vi "seriellTest.vi"() -> ()   [LabVIEW 2017]
uses:
  <vilib>/Utility/error.llb/Error Cluster From Error Code.vi
  <vilib>/rvi/errors/niLvFpgaAdjustHostInterfaceError.vi
  <vilib>/FPGAPlugInAG/cRIO-9035/niLvFpga_Close_cRIO-9035.vi
  <vilib>/rvi/interface/nirviMethod/nirviMethod.xnode
  FPGA Bitfiles/HAGAR-V_FPGATargetECD_FPGA-ProgrammECD_LbBtUh8SPQY.lvbitx
  FPGA_ECD/FPGA-Programm_ECD.vi
  <vilib>/rvi/interface/nirviReadWriteControl/nirviReadWriteControl.xnode
  <vilib>/rvi/interface/nirviCloseFPGA/nirviCloseFPGA.xnode
  <vilib>/FPGAPlugInAG/cRIO-9035/niLvFpga_ReadFifo_cRIO-9035.vi
  <vilib>/rvi/errors/niLvFpgaMergeErrorWithErrorCode.vi
  <vilib>/FPGAPlugInAG/cRIO-9035/niLvFpga_WriteFifo_cRIO-9035.vi
  NiFpgaLv.dll
panel:
  out "Angehängtes Array":i32[](array[numeric])
  in  "senden":bool
  in  "String":string
  out "Verknüpfter String":string
  out "error out":errorcluster
  in  "Stopp":bool
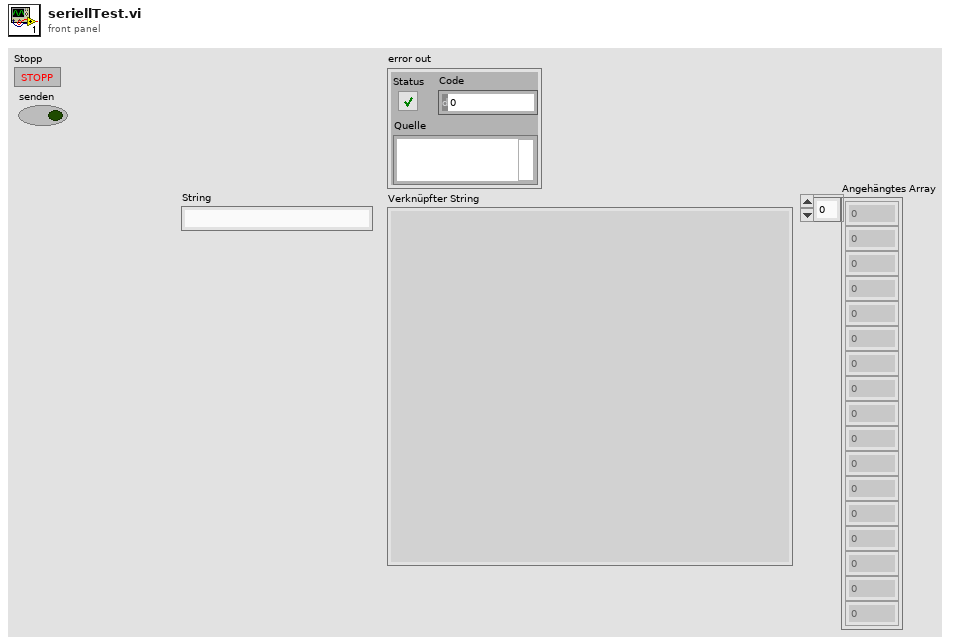
[diagram p1: front panel]
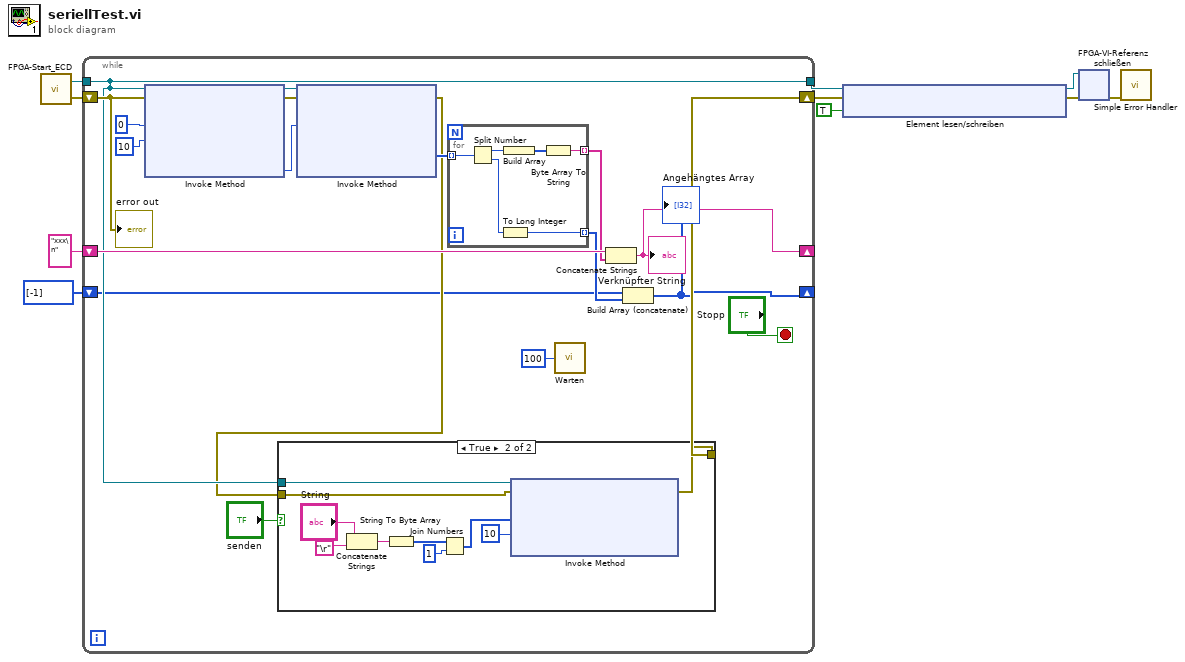
[diagram p0: block diagram]
diagram:
  n1 = call "FPGA-Start_ECD.vi"() -> ("error out"=w10:errorcluster, "FPGA-VI-Referenz (Ausgang)"=w1:refnum<k20>)  [unwired: 2 in]
  n2 = while {
    tunnel: w1 -> [w18]
    shift-right: [w16] -> w8
    shift-left: w10 -> [w24]
    tunnel: [w18] -> w9
    shift-right: [w19] -> _
    shift-left: "xxx\n" -> [w21]
    shift-right: [w13] -> _
    shift-left: i32[] [-1] -> [w12]
    stop <- "Stopp" stop-if-true
    n3 = xnode "Invoke Method"("FPGA-VI-Referenz (Eingang)"=w18, "Fehler (Eingang)"=w24, "Anzahl der Elemente"=u32 0 ("Number of Elements"), "Timeout (ms)"=10) -> ("FPGA-VI-Referenz (Ausgang)"=w26:refnum<k20>, "Fehler (Ausgang)"=w25:errorcluster, "Verbleibende Elemente"=w28:u32)  [unwired: 1 out]
    n4 = xnode "Invoke Method"("FPGA-VI-Referenz (Eingang)"=w26, "Fehler (Eingang)"=w25, "Anzahl der Elemente"=w28) -> ("Fehler (Ausgang)"=w17:errorcluster, "Daten"=w22:u16[])  [unwired: 1 in, 2 out]
    n5 = case shown="True" "senden" {
      tunnel: w18 -> [_ w34]
      tunnel: w17 -> [w30 w33]
      tunnel: [w30 w32] -> w16
      frame False {
      }
      frame True {
        n6 = Concatenate Strings("String", "\r") -> (w35:string)
        n7 = String To Byte Array(string=w35) -> (unsigned byte array=w40:u8[])
        n8 = Join Numbers(hi=w40, lo=u8 1) -> ((hi.lo)=w38:u16[])
        n9 = xnode "Invoke Method"("FPGA-VI-Referenz (Eingang)"=w34, "Fehler (Eingang)"=w33, "Daten"=w38, "Timeout (ms)"=10) -> ("Fehler (Ausgang)"=w32:errorcluster)  [unwired: 2 out]
      }
    }
    n10 = for {
      tunnel: w22 -> [w43] mode=indexing
      tunnel: [w42] -> w20 mode=indexing
      tunnel: [w41] -> w14 mode=indexing
      n11 = Split Number(x=w43) -> (hi(x)=w46:u8, lo(x)=w44:u8)
      n12 = To Long Integer(number=w44) -> (32bit integer=w41:i32)
      n13 = Build Array(w46) -> (w45:u8[])
      n14 = Byte Array To String(unsigned byte array=w45) -> (string=w42:string)
    }
    n15 = call "Warten"("Count(mSec)"=u32 100) -> ()  [unwired: 1 out]
    n16 = Concatenate Strings(w21, w20) -> (w19:string)
    "Verknüpfter String" <- w19
    n17 = Build Array (concatenate)(w12, w14) -> (w13:i32[])
    "Angehängtes Array" <- w13
    "error out" <- w24
  }
  n18 = xnode "Element lesen/schreiben"("FPGA-VI-Referenz (Eingang)"=w9, "Fehler (Eingang)"=w8, "global stop"=TRUE) -> ("FPGA-VI-Referenz (Ausgang)"=w6:refnum<k20>, "Fehler (Ausgang)"=w5:errorcluster)
  n19 = xnode "FPGA-VI-Referenz schließen"("FPGA-VI-Referenz (Eingang)"=w6, "Fehler (Eingang)"=w5) -> ("Fehler (Ausgang)"=w4:errorcluster)
  n20 = call <vilib>:"Simple Error Handler.vi"("error in (no error)"=w4) -> ()  [unwired: 4 in, 5 out]
